vi "BwCoeffSingleChanTemplate.vi"(0 "cutoff":dbl=2.0 format="%#_6p", 9 "sample rate":dbl=50000.0 format="%#_6p", 11 "error in (no error)":errorcluster) -> (4 "scaled coefficients":i32[](array[numeric]), 15 "error out":errorcluster)   [LabVIEW 2017, in "NI_FpgaMspHost.lvlib"]
doc: "This VI designs a Butterworth filter, then quantizes and formats the coefficients into 32-bit integers for use by the Butterworth Filter VI on the FPGA.\n\nThe user is responsible for ensuring that the configuration is valid. The following restrictions apply:\nCutoff frequency must meet Nyquist criterion.\nMultichannel filters are restricted to 2nd order.\nFilter order and type cannot be changed at run-time."
uses:
  <vilib>/rvi/Analysis/host/Public/NI_FpgaMspHost.lvlib
  <vilib>/rvi/Analysis/host/Butterworth/config/Butterworth Filter Order.ctl
  <vilib>/rvi/Analysis/host/Butterworth/config/Butterworth Filter Type.ctl
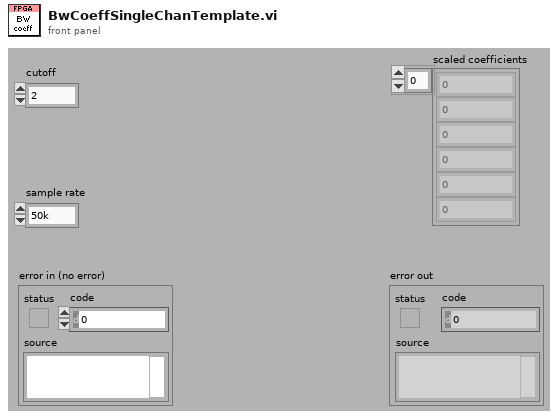
[diagram p1: front panel]
types:
  T1 = typedef "NI_FpgaMspHost.lvlib/Butterworth Filter Type.ctl" = u16
  T2 = typedef "NI_FpgaMspHost.lvlib/Butterworth Filter Order.ctl" = i32
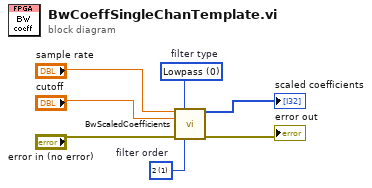
[diagram p0: block diagram]
diagram:
  w4 = T1 0 items=["Lowpass", "Highpass"]  # filter type
  w5 = T2 1 items=["1", "2", "4"]  # filter order
  n1 = call <vilib>:"BwScaledCoefficients.vi"("sample rate (S/s)"="sample rate", "filter type"=w4, "cutoff frequency (Hz)"="cutoff", "error in (no error)"="error in (no error)", "filter order"=w5) -> ("scaled coefficients"=→"scaled coefficients":i32[], "error out"=→"error out":errorcluster)  [unwired: 9 out]
